vi "Untitled 3.vi"(11 "Joystick Value":dbl) -> ()   [LabVIEW 2019]
panel:
  out "Motor Power":dbl
  in  "Multiplier":dbl
  in  "Dead Zone":dbl=0.4 format="%#_13g"
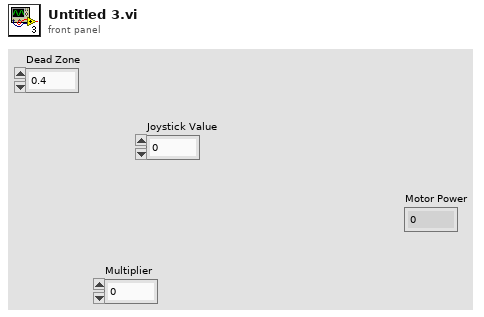
[diagram p1: front panel]
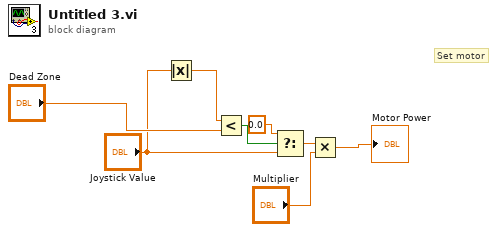
[diagram p0: block diagram]
diagram:
  # "Set motor"
  n1 = Absolute Value(x="Joystick Value") -> (abs(x)=w8:dbl)
  n2 = Less?(x=w8, y="Dead Zone") -> (x < y?=w6:bool)
  n3 = Select(t=0.0, s=w6, f="Joystick Value") -> (s? t:f=w2:dbl)
  n4 = Multiply(x=w2, y="Multiplier") -> (x*y=→"Motor Power":dbl)
